vi "My Theory.vi"(11 "condition":bool) -> (0 "error out":errorcluster)   [LabVIEW 2017]
uses:
  Assertion/Assertion.lvlib
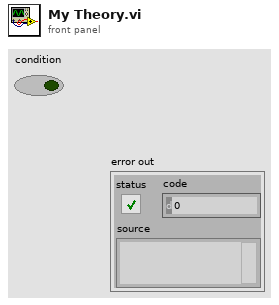
[diagram p1: front panel]
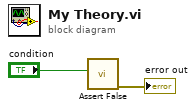
[diagram p0: block diagram]
diagram:
  n1 = call "Assert False.vi"("Condition"="condition") -> ("error out"=→"error out":errorcluster)  [unwired: 10 in]
